vi "LV FPGA Serial Read Write.vi"(0 "Transmit":refnum<k21>="Port4/DIO7", 5 "Receive":refnum<k21>="Port4/DIO8", 7 "baud rate (9600)":u32=9600, 9 "data bits (8)":i32=8 min=5 max=8 step=1, 11 "parity (0:none)":enum16{"None", "Odd", "Even", "Mark", "Space"}(ring), 12 "stop bits (10: 1 bit)":u16(ring)=10 items=["1.0"=10, "1.5"=15, "2.0"=20], 13 "Invert Polarity?":bool) -> ()   [LabVIEW 2009]
uses:
  <vilib>/eio/EIOMethodNode/EIOMethodNode.xnode
  <vilib>/rvi/eio/nirviEIOMethodImplementation/nirviEIOMethodImplementation.xnode
  <vilib>/rvi/eio/common/nirviEmuTemplateMethod_noerrors.vi
  <vilib>/rvi/eio/common/nirviEmuClasses.ctl
  <vilib>/eio/EIONode/EIONode.xnode
  <vilib>/rvi/eio/nirviEIOImplementation/nirviEIOImplementation.xnode
  Instance           1 27Saved   LV FPGA Serial Read .vi
  Instance           2 27Saved   LV FPGA Serial Read .vi
  Instance           3 27Saved   LV FPGA Serial Read .vi
  Instance           6 27Saved   LV FPGA Serial Read .vi
panel:
  out "Pin Input":bool
  out "Read Element":u8
  in  "Write Element":u8
  out "Read: Transmission Error":bool
  in  "stop":bool
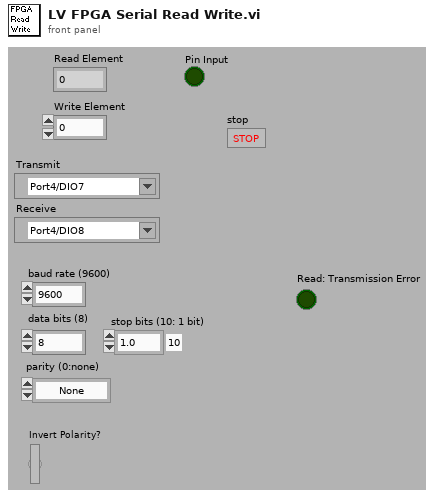
[diagram p1: front panel]
types:
  T1 = typedef "nirviEmuClasses.ctl" = enum16{"IO Read", "IO Write", "Method", "Property Read", "Property Write"}
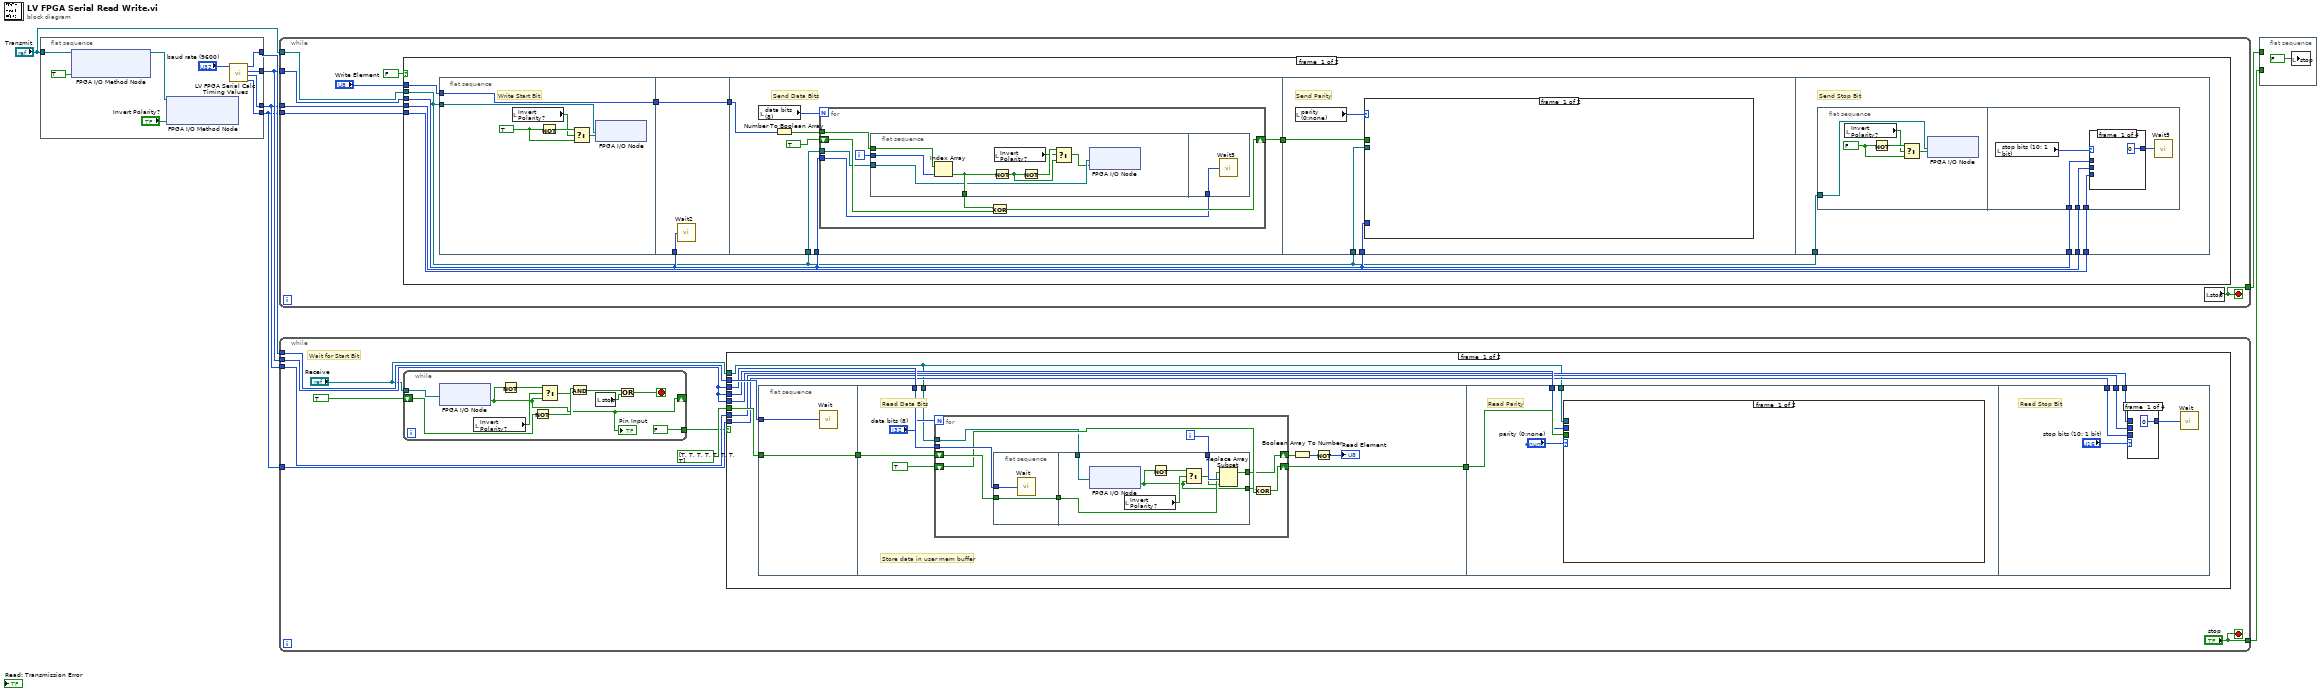
[diagram p0: block diagram]
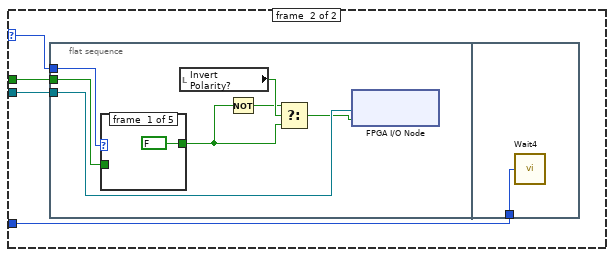
[diagram p2: hidden frame]
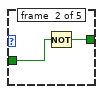
[diagram p3: hidden frame]
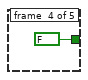
[diagram p5: hidden frame]
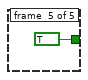
[diagram p6: hidden frame]
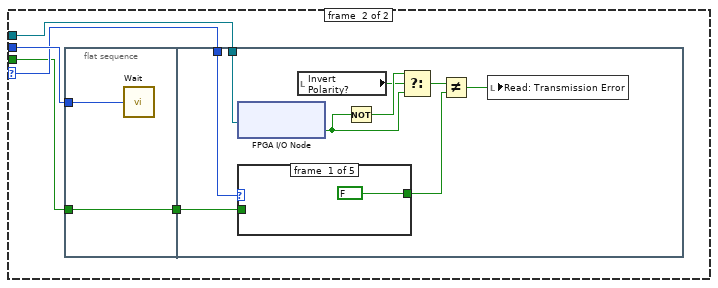
[diagram p11: hidden frame]
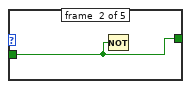
[diagram p12: hidden frame]
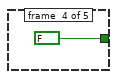
[diagram p14: hidden frame]
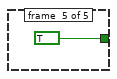
[diagram p15: hidden frame]
diagram:
  n1 = flat-sequence {
    tunnel: [w12] -> w6
    tunnel: [w15] -> w7
    tunnel: [w14] -> w5
    tunnel: [w13] -> w4
    tunnel: "Transmit" -> [w10]
    frame #0 {
      n2 = xnode "FPGA I/O Method Node"("FPGA I/O In"=w10, "Enable"=TRUE ("Digital Enable")) -> ("FPGA I/O Out"=w9:refnum<k21>)
      n3 = xnode "FPGA I/O Method Node"("FPGA I/O In"=w9, "Data"="Invert Polarity?") -> ()  [unwired: 1 out]
      n4 = call "LV FPGA Serial Calc Timing Values.vi"("baud rate (1000000)"="baud rate (9600)") -> ("Two Bit"=w13:u32, "One and Half Bit"=w14:u32, "One Bit"=w12:u32, "Half Bit"=w15:u32)  [unwired: 1 in, 2 out]
    }
  }
  n5 = while {
    tunnel: w4 -> [w45]
    tunnel: w5 -> [w44]
    tunnel: w6 -> [w43]
    tunnel: "Transmit" -> [w42]
    tunnel: [w41] -> w1
    stop <- w41 stop-if-true
    n6 = case shown="False" FALSE {
      tunnel: w45 -> [w50 _]
      tunnel: w44 -> [w49 _]
      tunnel: w43 -> [w48 _]
      tunnel: w42 -> [w47 _]
      tunnel: "Write Element" -> [w46 _]
      frame #0 {
        n7 = flat-sequence {
          tunnel: w47 -> [w59]
          tunnel: w46 -> [w54]
          tunnel: [w54] -> w53
          tunnel: w48 -> [w74]
          tunnel: [w73] -> w52
          tunnel: w53 -> [w73]
          tunnel: w48 -> [w81]
          tunnel: [w79] -> w51
          tunnel: w47 -> [w76]
          tunnel: w52 -> [w75]
          tunnel: w48 -> [w113]
          tunnel: w51 -> [w114]
          tunnel: w47 -> [w111]
          tunnel: w48 -> [w149]
          tunnel: w49 -> [w148]
          tunnel: w50 -> [w147]
          tunnel: w47 -> [w146]
          frame #0 {
            w57 = TRUE
            # "Write Start Bit"
            n8 = local read "Invert Polarity?"() -> (w56:bool)
            n9 = Not(x=w57) -> (.not. x?=w58:bool)
            n10 = Select(t=w58, s=w56, f=w57) -> (s? t:f=w55:bool)
            n11 = xnode "FPGA I/O Node"("I/O Item"=w55, "FPGA I/O In"=w59) -> ()  [unwired: 1 out]
          }
          frame #1 {
            n12 = call "Wait2"("Count(Ticks)"=w74) -> ()  [unwired: 1 out]
          }
          frame #2 {
            # "Send Data Bits"
            n13 = local read "data bits (8)"() -> (w77:i32)
            n14 = Number To Boolean Array(number=w75) -> (Boolean array=w78:bool[])
            n15 = for {
              N: w77 -> [_]
              tunnel: w81 -> [w85]
              shift-right: [w88] -> w79
              shift-left: TRUE -> [w87]
              tunnel: w78 -> [w84]
              tunnel: w76 -> [w82]
              i -> [w86]
              n16 = flat-sequence {
                tunnel: w86 -> [w96]
                tunnel: w84 -> [w95]
                tunnel: [w94] -> w83
                tunnel: w82 -> [w93]
                tunnel: w85 -> [w110]
                frame #0 {
                  n17 = Index Array(array=w95, index=w96) -> (element=w94:bool)
                  n18 = Not(x=w94) -> (.not. x?=w91:bool)
                  n19 = local read "Invert Polarity?"() -> (w90:bool)
                  n20 = Not(x=w91) -> (.not. x?=w92:bool)
                  n21 = Select(t=w92, s=w90, f=w91) -> (s? t:f=w89:bool)
                  n22 = xnode "FPGA I/O Node"("I/O Item"=w89, "FPGA I/O In"=w93) -> ()  [unwired: 1 out]
                }
                frame #1 {
                  n23 = call "Wait3"("Count(Ticks)"=w110) -> ()  [unwired: 1 out]
                }
              }
              n24 = Exclusive Or(1:w87, 2:w83) -> (0:w88:bool)
            }
          }
          frame #3 {
            # "Send Parity"
            n25 = local read "parity (0:none)"() -> (w112:enum16{"None", "Odd", "Even", "Mark", "Space"})
            n26 = case shown="\"Odd\", Default" w112 {
              selector: w112 -> [_ w118]
              tunnel: w114 -> [_ w117]
              tunnel: w113 -> [_ w116]
              tunnel: w111 -> [_ w115]
              frame #0 {
              }
              frame #1 {
                n27 = flat-sequence {
                  tunnel: w117 -> [w124]
                  tunnel: w118 -> [w125]
                  tunnel: w115 -> [w123]
                  tunnel: w116 -> [w145]
                  frame #0 {
                    n28 = case shown="\"Even\"" w125 {
                      tunnel: w124 -> [_ w141 w142 _ _]
                      tunnel: [FALSE ("y") w140 w142 FALSE ("y") TRUE ("y")] -> w120
                      frame #0 {
                      }
                      frame #1 {
                        n29 = Not(x=w141) -> (.not. x?=w140:bool)
                      }
                      frame #2 {
                      }
                      frame #3 {
                      }
                      frame #4 {
                      }
                    }
                    n30 = local read "Invert Polarity?"() -> (w122:bool)
                    n31 = Not(x=w120) -> (.not. x?=w121:bool)
                    n32 = Select(t=w121, s=w122, f=w120) -> (s? t:f=w119:bool)
                    n33 = xnode "FPGA I/O Node"("I/O Item"=w119, "FPGA I/O In"=w123) -> ()  [unwired: 1 out]
                  }
                  frame #1 {
                    n34 = call "Wait4"("Count(Ticks)"=w145) -> ()  [unwired: 1 out]
                  }
                }
              }
            }
          }
          frame #4 {
            # "Send Stop Bit"
            n35 = flat-sequence {
              tunnel: w146 -> [w154]
              tunnel: w149 -> [w172]
              tunnel: w148 -> [w171]
              tunnel: w147 -> [w170]
              frame #0 {
                w152 = FALSE
                n36 = local read "Invert Polarity?"() -> (w151:bool)
                n37 = Not(x=w152) -> (.not. x?=w153:bool)
                n38 = Select(t=w153, s=w151, f=w152) -> (s? t:f=w150:bool)
                n39 = xnode "FPGA I/O Node"("I/O Item"=w150, "FPGA I/O In"=w154) -> ()  [unwired: 1 out]
              }
              frame #1 {
                n40 = local read "stop bits (10: 1 bit)"() -> (w168:u16)
                n41 = case shown="20" w168 {
                  tunnel: w172 -> [_ w174 _ _]
                  tunnel: w171 -> [_ _ w175 _]
                  tunnel: w170 -> [_ _ _ w176]
                  tunnel: [u32 0 ("One Bit") w174 w175 w176] -> w169
                  frame #0 {
                  }
                  frame #1 {
                  }
                  frame #2 {
                  }
                  frame #3 {
                  }
                }
                n42 = call "Wait5"("Count(Ticks)"=w169) -> ()  [unwired: 1 out]
              }
            }
          }
        }
      }
      frame #1 {
      }
    }
    n43 = local read "stop"() -> (w41:bool)
  }
  n44 = while {
    tunnel: w4 -> [w184]
    tunnel: w5 -> [w183]
    tunnel: w6 -> [w182]
    tunnel: w7 -> [w181]
    tunnel: ["stop"] -> w2
    stop <- "stop" stop-if-true
    # "Wait for Start Bit"
    n45 = while {
      tunnel: [FALSE] -> w180
      shift-right: [w186] -> _
      shift-left: TRUE -> [w195]
      tunnel: "Receive" -> [w190]
      stop <- w191 stop-if-true
      n46 = xnode "FPGA I/O Node"("FPGA I/O In"=w190) -> ("I/O Item"=w186:bool)  [unwired: 1 out]
      "Pin Input" <- w186
      n47 = local read "Invert Polarity?"() -> (w188:bool)
      n48 = Not(x=w186) -> (.not. x?=w189:bool)
      n49 = Not(x=w195) -> (.not. x?=w194:bool)
      n50 = Select(t=w189, s=w188, f=w186) -> (s? t:f=w187:bool)
      n51 = And(x=w194, y=w187) -> (x .and. y?=w192:bool)
      n52 = local read "stop"() -> (w193:bool)
      n53 = Or(x=w192, y=w193) -> (x .or. y?=w191:bool)
    }
    n54 = case shown="False" w180 {
      tunnel: bool[] [TRUE, TRUE, TRUE, TRUE, TRUE, TRUE, TRUE, TRUE] -> [w226 _]
      tunnel: w181 -> [w225 _]
      tunnel: w182 -> [w224 _]
      tunnel: w182 -> [w223 _]
      tunnel: w182 -> [w222 _]
      tunnel: w183 -> [w221 _]
      tunnel: w184 -> [w220 _]
      tunnel: "Receive" -> [w218 _]
      frame #0 {
        n55 = flat-sequence {
          tunnel: [w229] -> w227
          tunnel: w226 -> [w229]
          tunnel: w225 -> [w228]
          tunnel: w227 -> [w238]
          tunnel: w224 -> [w237]
          tunnel: [w233] -> w219
          tunnel: w218 -> [w231]
          tunnel: w223 -> [w280]
          tunnel: w219 -> [w282]
          tunnel: w218 -> [w279]
          tunnel: w222 -> [w328]
          tunnel: w221 -> [w327]
          tunnel: w220 -> [w326]
          frame #0 {
            n56 = call "Wait"("Count(Ticks)"=w228) -> ()  [unwired: 1 out]
          }
          frame #1 {
            # "Store data in user mem buffer"
            # "Read Data Bits"
            n57 = for {
              N: "data bits (8)" -> [_]
              shift-right: [w241] -> w236
              shift-left: w238 -> [w247]
              tunnel: w237 -> [w245]
              shift-right: [w244] -> w233
              shift-left: TRUE -> [w243]
              tunnel: w231 -> [w239]
              i -> [w240]
              n58 = flat-sequence {
                tunnel: w247 -> [w249]
                tunnel: [w249] -> w246
                tunnel: w245 -> [w248]
                tunnel: w240 -> [w257]
                tunnel: w246 -> [w256]
                tunnel: [w255] -> w241
                tunnel: [w250] -> w242
                tunnel: w239 -> [w254]
                frame #0 {
                  n59 = call "Wait"("Count(Ticks)"=w248) -> ()  [unwired: 1 out]
                }
                frame #1 {
                  n60 = xnode "FPGA I/O Node"("FPGA I/O In"=w254) -> ("I/O Item"=w250:bool)  [unwired: 1 out]
                  n61 = local read "Invert Polarity?"() -> (w253:bool)
                  n62 = Not(x=w250) -> (.not. x?=w252:bool)
                  n63 = Select(t=w252, s=w253, f=w250) -> (s? t:f=w251:bool)
                  n64 = Replace Array Subset(array=w256, new element=w251, index=w257) -> (w255:bool[])
                }
              }
              n65 = Exclusive Or(1:w243, 2:w242) -> (0:w244:bool)
            }
            n66 = Boolean Array To Number(Boolean array=w236) -> (number=w235:u8)
            n67 = Not(x=w235) -> (.not. x?=→"Read Element":u8)
          }
          frame #2 {
            # "Read Parity"
            n68 = case shown="\"Odd\", Default" "parity (0:none)" {
              selector: "parity (0:none)" -> [_ w286]
              tunnel: w282 -> [_ w284]
              tunnel: w280 -> [_ w287]
              tunnel: w279 -> [_ w283]
              frame #0 {
              }
              frame #1 {
                n69 = flat-sequence {
                  tunnel: w287 -> [w289]
                  tunnel: [w288] -> w285
                  tunnel: w284 -> [w288]
                  tunnel: w286 -> [w298]
                  tunnel: w285 -> [w296]
                  tunnel: w283 -> [w294]
                  frame #0 {
                    n70 = call "Wait"("Count(Ticks)"=w289) -> ()  [unwired: 1 out]
                  }
                  frame #1 {
                    n71 = xnode "FPGA I/O Node"("FPGA I/O In"=w294) -> ("I/O Item"=w291:bool)  [unwired: 1 out]
                    n72 = case shown="\"None\"" w298 {
                      tunnel: w296 -> [_ w321 w322 _ _]
                      tunnel: [FALSE ("y") w321 w322 FALSE ("y") TRUE ("y")] -> w297
                      frame #0 {
                      }
                      frame #1 {
                        n73 = Not(x=w321) -> ()  [unwired: 1 out]
                      }
                      frame #2 {
                      }
                      frame #3 {
                      }
                      frame #4 {
                      }
                    }
                    n74 = local read "Invert Polarity?"() -> (w292:bool)
                    n75 = Not(x=w291) -> (.not. x?=w293:bool)
                    n76 = Select(t=w293, s=w292, f=w291) -> (s? t:f=w290:bool)
                    n77 = Not Equal?(x=w290, y=w297) -> (x != y?=w295:bool)
                    n78 = local write "Read: Transmission Error"(w295) -> ()
                  }
                }
              }
            }
          }
          frame #3 {
            # "Read Stop Bit"
            n79 = case shown="10" "stop bits (10: 1 bit)" {
              tunnel: w328 -> [_ w331 _ _]
              tunnel: w327 -> [_ _ w332 _]
              tunnel: w326 -> [_ _ _ w333]
              tunnel: [u32 0 ("One Bit") w331 w332 w333] -> w325
              frame #0 {
              }
              frame #1 {
              }
              frame #2 {
              }
              frame #3 {
              }
            }
            n80 = call "Wait"("Count(Ticks)"=w325) -> ()  [unwired: 1 out]
          }
        }
      }
      frame #1 {
      }
    }
  }
  n81 = flat-sequence {
    tunnel: w2 -> [_]
    tunnel: w1 -> [_]
    frame #0 {
      n82 = local write "stop"(FALSE ("stop")) -> ()
    }
  }
